vi "Start Device.vi"(8 "error in (no error)":errorcluster, 10 "device":string, 11 "Device Manager in":refnum<class "Device Manager.lvclass">) -> (0 "error out":errorcluster, 3 "Device Manager out":refnum<class "Device Manager.lvclass">)   [LabVIEW 2020, in "Device Manager.lvclass"]
uses:
  Device Manager.lvclass
  Device/Device Messages/Start Action Msg/Start Action Msg.lvclass
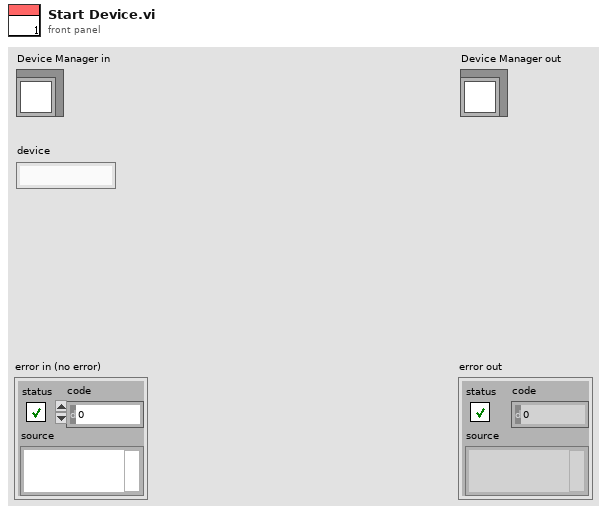
[diagram p1: front panel]
types:
  T1 = map{string, refnum<class "Message Enqueuer.lvclass">}
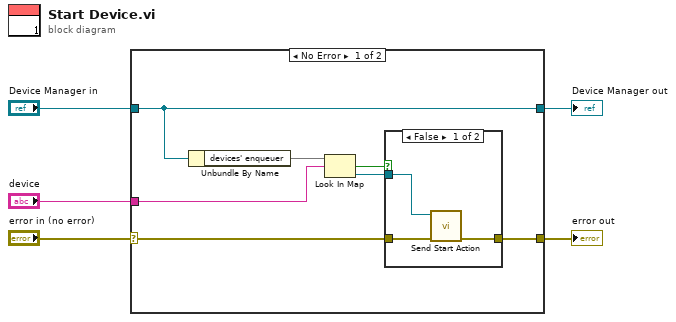
[diagram p0: block diagram]
diagram:
  n1 = case shown="No Error" "error in (no error)" {
    selector: "error in (no error)" -> [w12 w18]
    tunnel: [w7 w18] -> w4
    tunnel: [w11 w17] -> w2
    tunnel: "Device Manager in" -> [w11 w17]
    tunnel: "device" -> [w9 _]
    frame No Error {
      n2 = Unbundle By Name(w11) -> ("devices' enqueuer"=w10:T1)
      n3 = Look In Map(map=w10, key=w9) -> (key not found?=w8:bool, value=w6:refnum<class "Message Enqueuer.lvclass">)  [unwired: 1 in]
      n4 = case shown="False" w8 {
        tunnel: w12 -> [w15 w16]
        tunnel: [w14 w16] -> w7
        tunnel: w6 -> [w13 _]
        frame False {
          n5 = call "Send Start Action.vi"("error in (no error)"=w15, "Message Enqueuer"=w13) -> ("error out"=w14:errorcluster)  [unwired: 8 in, 1 out]
        }
        frame True {
        }
      }
    }
    frame Error {
    }
  }
  "error out" <- w4
  "Device Manager out" <- w2
